vi "Build meas status string.vi"(11 "Cell details cluster in":T1) -> (3 "Measurement status":string)   [LabVIEW 2011]
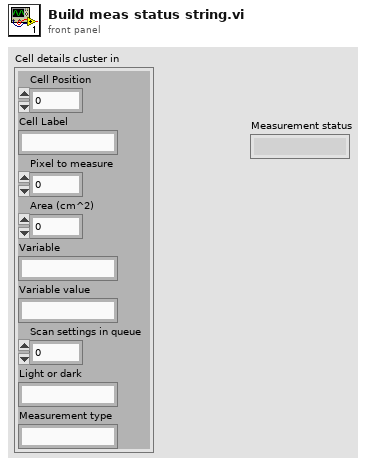
[diagram p1: front panel]
types:
  T1 = cluster{"Cell Position":i32, "Cell Label":string, "Pixel to measure":u16, "Area (cm^2)":dbl, "Variable":string, "Variable value":string, "Scan settings in queue":u16, "Light or dark":string, "Measurement type":string}
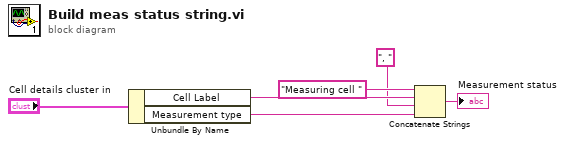
[diagram p0: block diagram]
diagram:
  n1 = Unbundle By Name("Cell details cluster in") -> ("Cell Label"=w4:string, "Measurement type"=w2:string)
  n2 = Concatenate Strings("Measuring cell " ("string"), w4, ", ", w2) -> (→"Measurement status":string)
